vi "DB Get Station Type.vi"(8 "error in (no error)":errorcluster) -> (0 "error out":errorcluster, 2 "Station Types":string[](array[string]))   [LabVIEW 2019, in "Control Experiment.lvclass"]
uses:
  Control Experiment.lvclass
  <userlib>/LevyLab/LV-Data/LV-Data.PG/LV-Data.PGSQL.lvclass
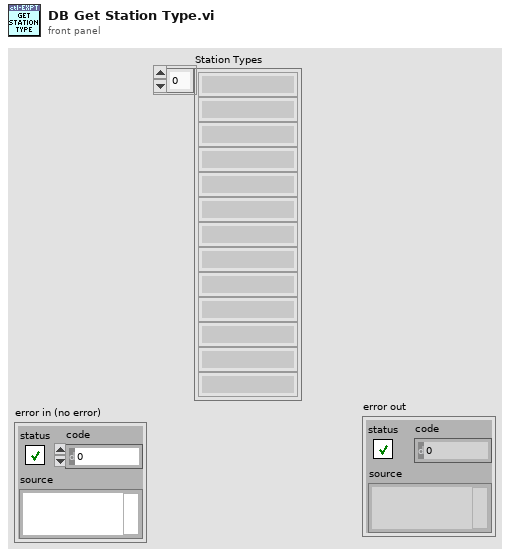
[diagram p1: front panel]
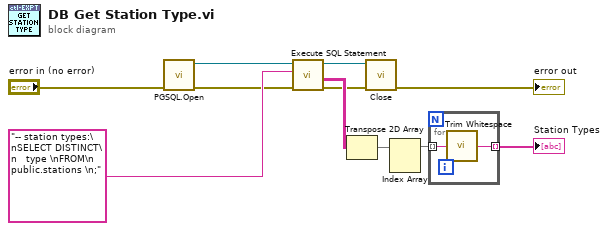
[diagram p0: block diagram]
diagram:
  n1 = call <userlib>:"PGSQL.Open.vi"("error in (no error)"="error in (no error)") -> ("error out"=w4:errorcluster, "Data.PG out"=w9:refnum<class "LV-Data.PGSQL.lvclass">)  [unwired: 9 in]
  n2 = call <userlib>:"Execute SQL Statement.vi"("error in (no error)"=w4, "SQL string"="-- station types:\nSELECT DISTINCT\n   type \nFROM\n   public.stations \n;" ("Address"), "Data.PGQL in"=w9) -> ("error out"=w3:errorcluster, "Result"=w7:string[][], "Data.PGSQL out"=w8:refnum<class "LV-Data.PGSQL.lvclass">)  [unwired: 6 in]
  n3 = Transpose 2D Array(2D array=w7) -> (transposed array=w1:string[][])
  n4 = call-dynamic "Close.vi"("error in (no error)"=w3, "Data.PG in"=w8) -> ("error out"=→"error out":errorcluster)  [unwired: 8 in, 1 out]
  n5 = Index Array(array=w1) -> (element=w6:string[])  [unwired: 2 in]
  n6 = for {
    tunnel: w6 -> [w13] mode=indexing
    tunnel: [w12] -> w11 mode=indexing
    n7 = call <vilib>:"Trim Whitespace.vi"("string"=w13) -> ("trimmed string"=w12:string)  [unwired: 1 in]
  }
  "Station Types" <- w11
